vi "sub_SDR_mod_stringToBPSK.vi"(11 "Input String":string) -> (3 "Array":i16[](array[numeric]))   [LabVIEW 2012]
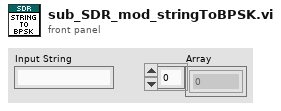
[diagram p1: front panel]
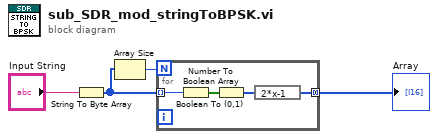
[diagram p0: block diagram]
diagram:
  n1 = String To Byte Array(string="Input String") -> (unsigned byte array=w3:u8[])
  n2 = Array Size(array=w3) -> (size(s)=w2:i32)
  n3 = for {
    N: w2 -> [_]
    tunnel: w3 -> [w8] mode=indexing
    tunnel: [w5] -> w4 mode=concatenating
    n4 = Number To Boolean Array(number=w8) -> (Boolean array=w7:bool[])
    n5 = Boolean To (0,1)(Boolean=w7) -> (0, 1=w6:i16[])
    n6 = expression code="2*x-1"(w6) -> (w5:i16[])
  }
  "Array" <- w4
